vi "试验判定 - 副本.vi"(7 "Result":refnum<vi>, 10 "判定参数":T1, 11 "XY曲线":cluster{"X":dbl[], "Y":dbl[]}[](array[cluster])) -> (2 "判定项长度":i32, 3 "OK？":bool)   [LabVIEW 2020]
uses:
  Global_Variable/Global.vi
  Global_Variable/A131258.vi
  <userlib>/_MGI/1D Array/MGI Average/MGI Average (DBL[]).vi
panel:
  out "逆向平均值":dbl
  out "正向平均值":dbl
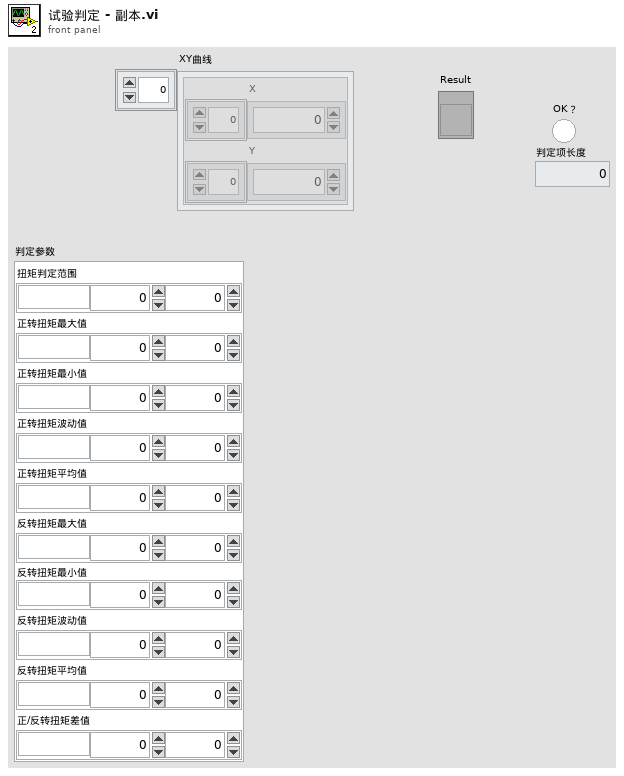
[diagram p1: front panel]
types:
  T1 = cluster{"扭矩判定范围":cluster{"单位":string, "下限":dbl, "上限":dbl}, "正转扭矩最大值":cluster{"单位":string, "下限":dbl, "上限":dbl}, "正转扭矩最小值":cluster{"单位":string, "下限":dbl, "上限":dbl}, "正转扭矩波动值":cluster{"单位":string, "下限":dbl, "上限":dbl}, "正转扭矩平均值":cluster{"单位":string, "下限":dbl, "上限":dbl}, "反转扭矩最大值":cluster{"单位":string, "下限":dbl, "上限":dbl}, "反转扭矩最小值":cluster{"单位":string, "下限":dbl, "上限":dbl}, "反转扭矩波动值":cluster{"单位":string, "下限":dbl, "上限":dbl}, "反转扭矩平均值":cluster{"单位":string, "下限":dbl, "上限":dbl}, "正/反转扭矩差值":cluster{"单位":string, "下限":dbl, "上限":dbl}}
  T2 = cluster{"左平均扭矩":cluster{"正转":dbl, "反转":dbl}, "左矩波动":cluster{"正转":dbl, "反转":dbl}, "左空载":cluster{"正转":dbl, "反转":dbl}, "右平均扭矩":cluster{"正转":dbl, "反转":dbl}, "右扭矩波动":cluster{"正转":dbl, "反转":dbl}, "右空载":cluster{"正转":dbl, "反转":dbl}, "扭矩对称":cluster{"左":dbl, "右":dbl}, "左零点漂移":cluster{"正":dbl, "反":dbl}, "右零点漂移":cluster{"正":dbl, "反":dbl}}
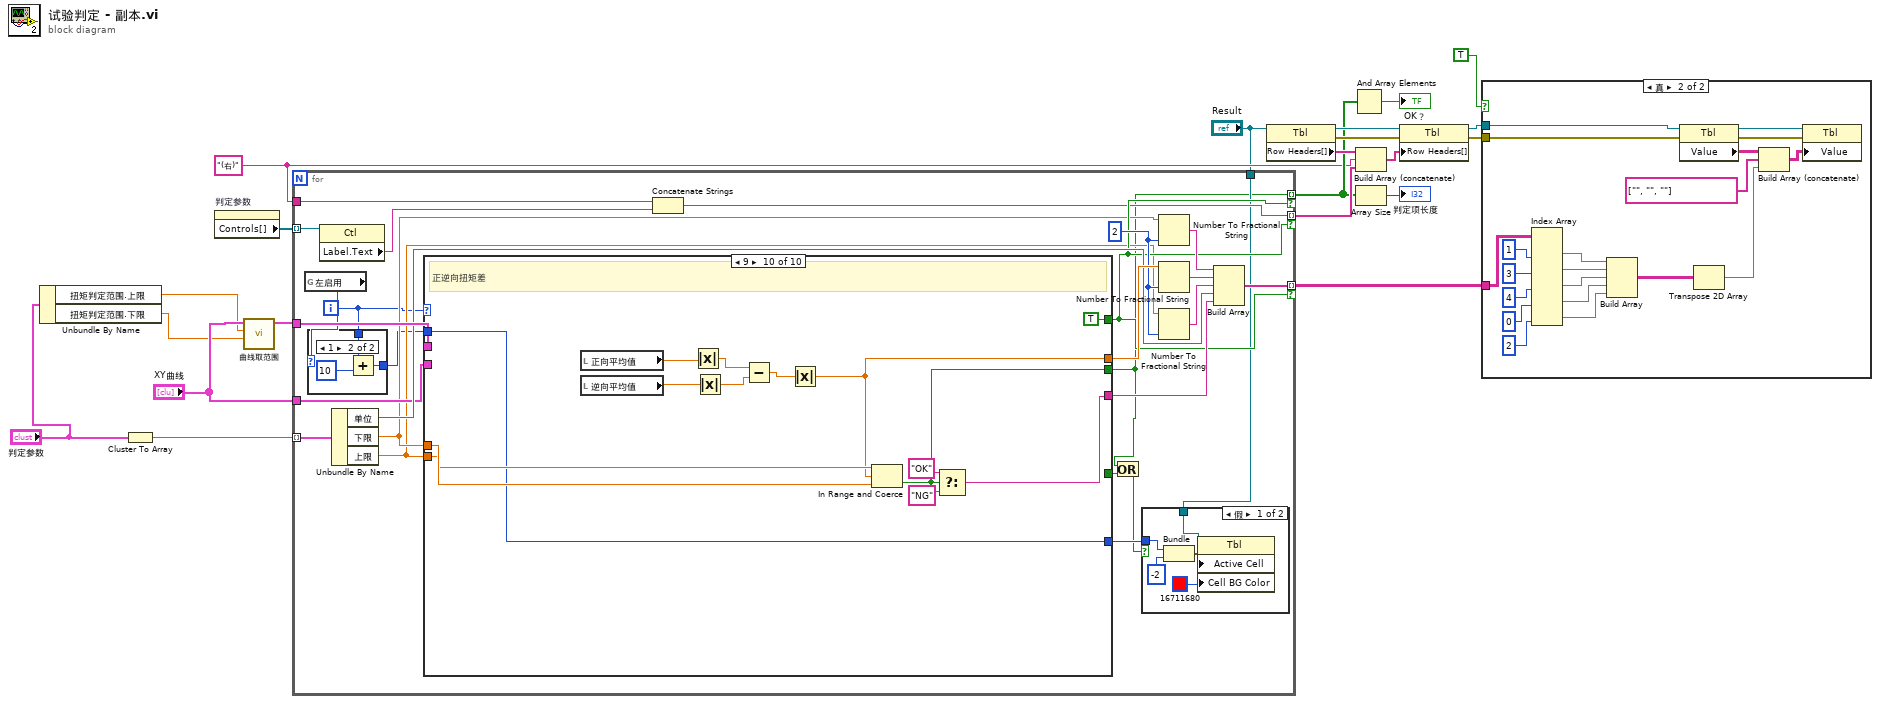
[diagram p0: block diagram]
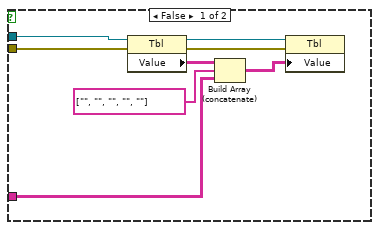
[diagram p2: hidden frame]
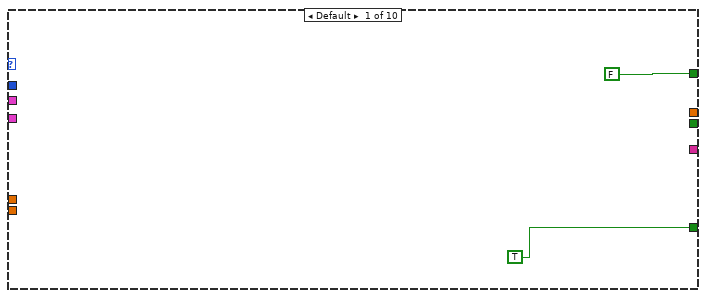
[diagram p5: hidden frame]
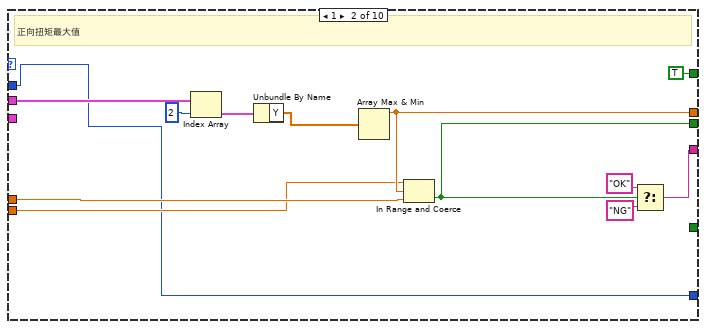
[diagram p6: hidden frame]
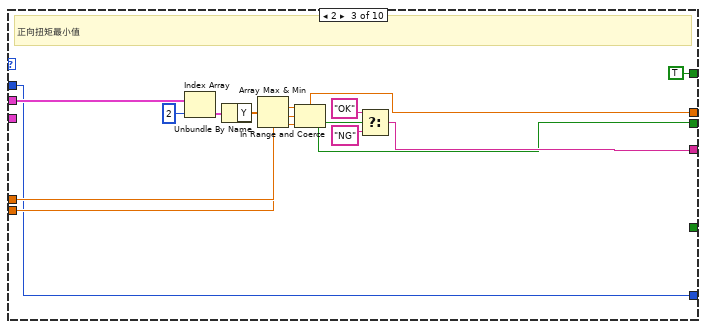
[diagram p7: hidden frame]
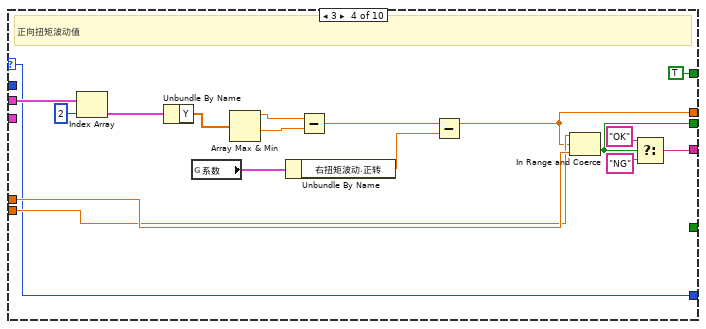
[diagram p8: hidden frame]
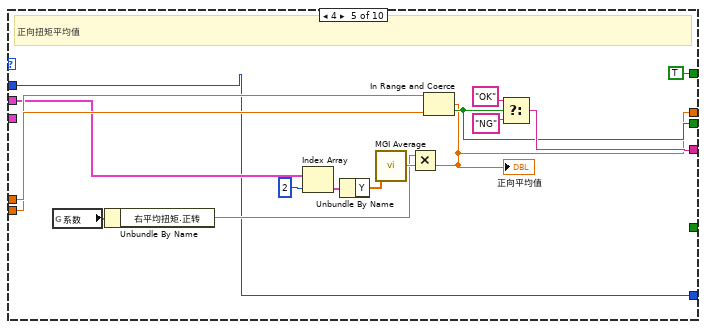
[diagram p9: hidden frame]
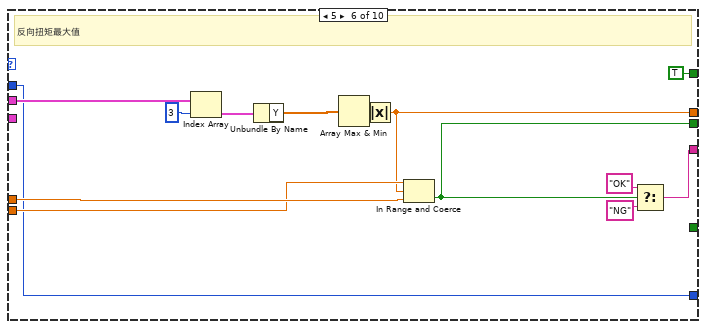
[diagram p10: hidden frame]
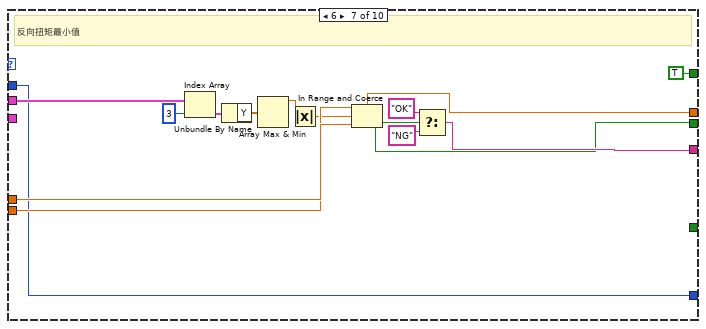
[diagram p11: hidden frame]
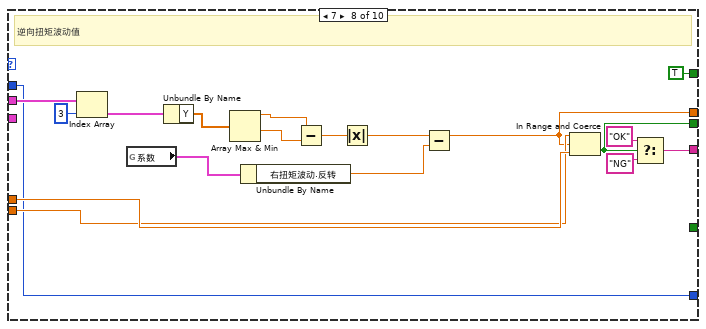
[diagram p12: hidden frame]
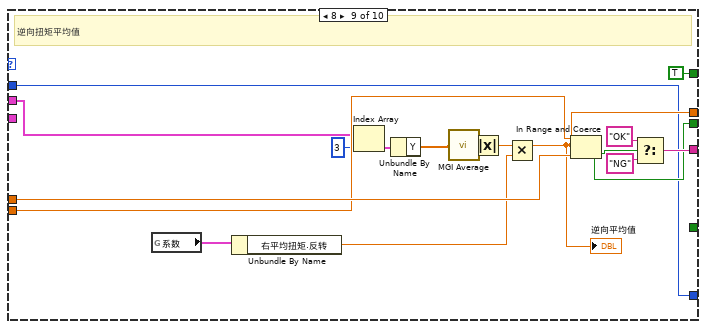
[diagram p13: hidden frame]
diagram:
  w7 = "(右)" ("Label.Text")
  n1 = Unbundle By Name("判定参数") -> ("扭矩判定范围.上限"=w2:dbl, "扭矩判定范围.下限"=w3:dbl)
  n2 = Cluster To Array(cluster="判定参数") -> (array=w21:cluster{"单位":string, "下限":dbl, "上限":dbl}[])
  n3 = property on="判定参数" class="Clust (严格)"() -> ("Controls[]"=w11:refnum<vi>[])  [unwired: 2 in, 2 out]
  n4 = call "曲线取范围.vi"("下限"=w3, "上限"=w2, "曲线In"="XY曲线") -> ("曲线Out"=w5:cluster{"X":dbl[], "Y":dbl[]}[])  [unwired: 8 in]
  n5 = for {
    tunnel: w21 -> [w47] mode=indexing
    tunnel: w11 -> [w46] mode=indexing
    tunnel: w5 -> [w44]
    tunnel: [w27] -> w9 mode=indexing if=w35
    tunnel: [w37] -> w12 mode=indexing if=w35
    tunnel: [w31] -> w14 mode=indexing if=w35
    tunnel: "XY曲线" -> [w34]
    tunnel: w7 -> [w30]
    tunnel: "Result" -> [w29]
    i -> [w24]
    w43 = i16 2 ("精度(6)")
    n6 = global read "Global.vi" "左启用"() -> (w22:i16)
    n7 = case shown="1" w22 {
      tunnel: w24 -> [w48 w50]
      tunnel: [w48 w49] -> w23
      frame 0, Default {
      }
      frame 1 {
        n8 = Add(x=w50, y=10) -> (x+y=w49:i32)
      }
    }
    n9 = property class="Ctl"(reference=w46) -> ("Label.Text"=w36:string)  [unwired: 1 in, 2 out]
    n10 = Unbundle By Name(w47) -> ("单位"=w38:string, "下限"=w33:dbl, "上限"=w32:dbl)
    n11 = case shown="9" w24 {
      selector: w24 -> [_ _ _ w85 _ _ _ _ _ _]
      tunnel: [_ w68 w76 w87 w105 w121 w135 w149 w168 w185] -> w45
      tunnel: w44 -> [_ w71 w84 w96 w112 w132 w146 w159 w176 _]
      tunnel: [_ w65 w80 w100 w116 w127 w142 w163 w180 w186] -> w39
      tunnel: [_ w60 w73 w89 w107 w120 w134 w151 w170 w184] -> w27
      tunnel: w33 -> [_ w64 w79 w99 w115 w126 w141 w162 w179 w193]
      tunnel: w32 -> [_ w63 w78 w98 w114 w125 w140 w161 w178 w192]
      tunnel: [FALSE TRUE TRUE TRUE TRUE TRUE TRUE TRUE TRUE TRUE] -> w35
      tunnel: w34 -> [_ _ _ _ _ _ _ _ _ _]
      tunnel: [_ w59 w72 w85 w103 w119 w133 w147 w166 w183] -> w28
      tunnel: [TRUE _ _ _ _ _ _ _ _ _] -> w25
      tunnel: w23 -> [_ w59 w72 _ w103 w119 w133 w147 w166 w183]
      frame Default {
      }
      frame 1 {
        # "正向扭矩最大值"
        n12 = Index Array(array=w71, index=2 ("索引")) -> (element=w69:cluster{"X":dbl[], "Y":dbl[]})
        n13 = Unbundle By Name(w69) -> ("Y"=w61:dbl[])
        n14 = Array Max & Min(array=w61) -> (max value=w68:dbl)  [unwired: 3 out]
        n15 = In Range and Coerce(upper limit=w63, x=w68, lower limit=w64) -> (In Range?=w60:bool)  [unwired: 1 out]
        n16 = Select(t="OK", s=w60, f="NG") -> (s? t:f=w65:string)
      }
      frame 2 {
        # "正向扭矩最小值"
        n17 = Index Array(array=w84, index=2 ("索引")) -> (element=w83:cluster{"X":dbl[], "Y":dbl[]})
        n18 = Unbundle By Name(w83) -> ("Y"=w75:dbl[])
        n19 = Array Max & Min(array=w75) -> (min value=w76:dbl)  [unwired: 3 out]
        n20 = In Range and Coerce(upper limit=w78, x=w76, lower limit=w79) -> (In Range?=w73:bool)  [unwired: 1 out]
        n21 = Select(t="OK", s=w73, f="NG") -> (s? t:f=w80:string)
      }
      frame 3 {
        # "正向扭矩波动值"
        n22 = Index Array(array=w96, index=2 ("索引")) -> (element=w95:cluster{"X":dbl[], "Y":dbl[]})
        n23 = Unbundle By Name(w95) -> ("Y"=w93:dbl[])
        n24 = global read "A131258.vi" "系数"() -> (w88:T2)
        n25 = Array Max & Min(array=w93) -> (max value=w92:dbl, min value=w91:dbl)  [unwired: 2 out]
        n26 = Unbundle By Name(w88) -> ("右扭矩波动.正转"=w86:dbl)
        n27 = Subtract(x=w92, y=w91) -> (x-y=w90:dbl)
        n28 = Subtract(x=w90, y=w86) -> (x-y=w87:dbl)
        n29 = In Range and Coerce(upper limit=w98, x=w87, lower limit=w99) -> (In Range?=w89:bool)  [unwired: 1 out]
        n30 = Select(t="OK", s=w89, f="NG") -> (s? t:f=w100:string)
      }
      frame 4 {
        # "正向扭矩平均值"
        n31 = global read "A131258.vi" "系数"() -> (w106:T2)
        n32 = Unbundle By Name(w106) -> ("右平均扭矩.正转"=w104:dbl)
        n33 = Index Array(array=w112, index=2 ("索引")) -> (element=w111:cluster{"X":dbl[], "Y":dbl[]})
        n34 = Unbundle By Name(w111) -> ("Y"=w108:dbl[])
        n35 = call-poly <userlib>:"MGI Average.vi"("Double[]"=w108) -> ("Average"=w109:dbl)  [unwired: 1 in]
        n36 = Multiply(x=w104, y=w109) -> (x*y=w105:dbl)
        "正向平均值" <- w105
        n37 = In Range and Coerce(upper limit=w114, x=w105, lower limit=w115) -> (In Range?=w107:bool)  [unwired: 1 out]
        n38 = Select(t="OK", s=w107, f="NG") -> (s? t:f=w116:string)
      }
      frame 5 {
        # "反向扭矩最大值"
        n39 = Index Array(array=w132, index=3 ("索引")) -> (element=w130:cluster{"X":dbl[], "Y":dbl[]})
        n40 = Unbundle By Name(w130) -> ("Y"=w123:dbl[])
        n41 = Array Max & Min(array=w123) -> (min value=w122:dbl)  [unwired: 3 out]
        n42 = Absolute Value(x=w122) -> (abs(x)=w121:dbl)
        n43 = In Range and Coerce(upper limit=w125, x=w121, lower limit=w126) -> (In Range?=w120:bool)  [unwired: 1 out]
        n44 = Select(t="OK", s=w120, f="NG") -> (s? t:f=w127:string)
      }
      frame 6 {
        # "反向扭矩最小值"
        n45 = Index Array(array=w146, index=3 ("索引")) -> (element=w145:cluster{"X":dbl[], "Y":dbl[]})
        n46 = Unbundle By Name(w145) -> ("Y"=w138:dbl[])
        n47 = Array Max & Min(array=w138) -> (max value=w136:dbl)  [unwired: 3 out]
        n48 = Absolute Value(x=w136) -> (abs(x)=w135:dbl)
        n49 = In Range and Coerce(upper limit=w140, x=w135, lower limit=w141) -> (In Range?=w134:bool)  [unwired: 1 out]
        n50 = Select(t="OK", s=w134, f="NG") -> (s? t:f=w142:string)
      }
      frame 7 {
        # "逆向扭矩波动值"
        n51 = Index Array(array=w159, index=3 ("索引")) -> (element=w158:cluster{"X":dbl[], "Y":dbl[]})
        n52 = global read "A131258.vi" "系数"() -> (w150:T2)
        n53 = Unbundle By Name(w158) -> ("Y"=w156:dbl[])
        n54 = Array Max & Min(array=w156) -> (max value=w155:dbl, min value=w154:dbl)  [unwired: 2 out]
        n55 = Unbundle By Name(w150) -> ("右扭矩波动.反转"=w148:dbl)
        n56 = Subtract(x=w155, y=w154) -> (x-y=w153:dbl)
        n57 = Absolute Value(x=w153) -> (abs(x)=w152:dbl)
        n58 = Subtract(x=w152, y=w148) -> (x-y=w149:dbl)
        n59 = In Range and Coerce(upper limit=w161, x=w149, lower limit=w162) -> (In Range?=w151:bool)  [unwired: 1 out]
        n60 = Select(t="OK", s=w151, f="NG") -> (s? t:f=w163:string)
      }
      frame 8 {
        # "逆向扭矩平均值"
        n61 = global read "A131258.vi" "系数"() -> (w169:T2)
        n62 = Unbundle By Name(w169) -> ("右平均扭矩.反转"=w167:dbl)
        n63 = Index Array(array=w176, index=3 ("索引")) -> (element=w175:cluster{"X":dbl[], "Y":dbl[]})
        n64 = Unbundle By Name(w175) -> ("Y"=w174:dbl[])
        n65 = call-poly <userlib>:"MGI Average.vi"("Double[]"=w174) -> ("Average"=w172:dbl)  [unwired: 1 in]
        n66 = Absolute Value(x=w172) -> (abs(x)=w171:dbl)
        n67 = Multiply(x=w171, y=w167) -> (x*y=w168:dbl)
        "逆向平均值" <- w168
        n68 = In Range and Coerce(upper limit=w178, x=w168, lower limit=w179) -> (In Range?=w170:bool)  [unwired: 1 out]
        n69 = Select(t="OK", s=w170, f="NG") -> (s? t:f=w180:string)
      }
      frame 9 {
        # "正逆向扭矩差"
        n70 = local read "正向平均值"() -> (w191:dbl)
        n71 = local read "逆向平均值"() -> (w190:dbl)
        n72 = Absolute Value(x=w191) -> (abs(x)=w189:dbl)
        n73 = Absolute Value(x=w190) -> (abs(x)=w188:dbl)
        n74 = Subtract(x=w189, y=w188) -> (x-y=w187:dbl)
        n75 = Absolute Value(x=w187) -> (abs(x)=w185:dbl)
        n76 = In Range and Coerce(upper limit=w192, x=w185, lower limit=w193) -> (In Range?=w184:bool)  [unwired: 1 out]
        n77 = Select(t="OK", s=w184, f="NG") -> (s? t:f=w186:string)
      }
    }
    n78 = Concatenate Strings(w30, w36) -> (w31:string)
    n79 = Or(x=w27, y=w25) -> (x .or. y?=w26:bool)
    n80 = case shown="假" w26 {
      tunnel: w29 -> [w56 _]
      tunnel: w28 -> [w52 _]
      frame False {
        n81 = Bundle(w52, -2) -> (w54:cluster{i32, i32})  [unwired: 1 in]
        n82 = property class="Tbl"(reference=w56, "Active Cell"=w54, "Cell BG Color"=u32 16711680 ("活动单元格:单元格背景色")) -> ()  [unwired: 1 in, 2 out]
      }
      frame True {
      }
    }
    n83 = Number To Fractional String(number=w33, precision (6)=w43) -> (F-format string=w42:string)  [unwired: 2 in]
    n84 = Number To Fractional String(number=w45, precision (6)=w43) -> (F-format string=w41:string)  [unwired: 2 in]
    n85 = Number To Fractional String(number=w32, precision (6)=w43) -> (F-format string=w40:string)  [unwired: 2 in]
    n86 = Build Array(w42, w41, w40, w38, w39) -> (w37:string[])
  }
  n87 = property class="Tbl"(reference="Result") -> (reference out=w16:refnum<vi>, error out=w19:errorcluster, "Row Headers[]"=w13:string[])  [unwired: 1 in]
  n88 = And Array Elements(Boolean array=w9) -> (logical AND=→"OK？":bool)
  n89 = Build Array (concatenate)(w13, w7, w14) -> (w15:string[])
  n90 = Array Size(array=w9) -> (size(s)=→"判定项长度":i32)
  n91 = property class="Tbl"(reference=w16, error in=w19, "Row Headers[]"=w15) -> (reference out=w17:refnum<vi>, error out=w18:errorcluster)
  n92 = case shown="真" TRUE {
    tunnel: w18 -> [w202 w222]
    tunnel: w17 -> [w199 w219]
    tunnel: w12 -> [w198 w217]
    frame False {
      n93 = property class="Tbl"(reference=w199, error in=w202) -> (reference out=w200:refnum<vi>, error out=w201:errorcluster, "Value"=w203:string[][])
      n94 = Build Array (concatenate)(w203, string[] ["", "", "", "", ""], w198) -> (w204:string[][])
      n95 = property class="Tbl"(reference=w200, error in=w201, "Value"=w204) -> ()  [unwired: 2 out]
    }
    frame True {
      n96 = Index Array(array=w217, index (col) #1=1 ("禁用的索引 (列)"), index (col) #2=3 ("索引 (列)"), index (col) #3=4 ("索引 (列)"), index (col) #4=0 ("索引 (列)"), index (col) #5=2 ("索引 (列)")) -> (element #1=w213:string[], element #2=w212:string[], element #3=w211:string[], element #4=w206:string[], element #5=w205:string[])  [unwired: 5 in]
      n97 = Build Array(w213, w212, w211, w206, w205) -> (w210:string[][])
      n98 = property class="Tbl"(reference=w219, error in=w222) -> (reference out=w220:refnum<vi>, error out=w221:errorcluster, "Value"=w223:string[][])
      n99 = Transpose 2D Array(2D array=w210) -> (transposed array=w209:string[][])
      n100 = Build Array (concatenate)(w223, string[] ["", "", ""], w209) -> (w224:string[][])
      n101 = property class="Tbl"(reference=w220, error in=w221, "Value"=w224) -> ()  [unwired: 2 out]
    }
  }
